vi "Get Tests for Key.vi"(8 "error in (no error)":errorcluster, 10 "Key":string, 11 "Test Event Storage in":refnum<class "Test Event Storage.lvclass">) -> (0 "error out":errorcluster, 2 "Test Events":T1[](array[typedef]), 3 "Test Event Storage out":refnum<class "Test Event Storage.lvclass">)   [LabVIEW 2009, in "Caraya.lvlib" / "Test Event Storage.lvclass"]
uses:
  Test Event Storage.lvclass
  Basic Test Manager/Assert Event Data.ctl
  Test Event Storage.lvclass/Test Event Storage.ctl
  Basic Test Manager/Basic Test Manager.lvclass
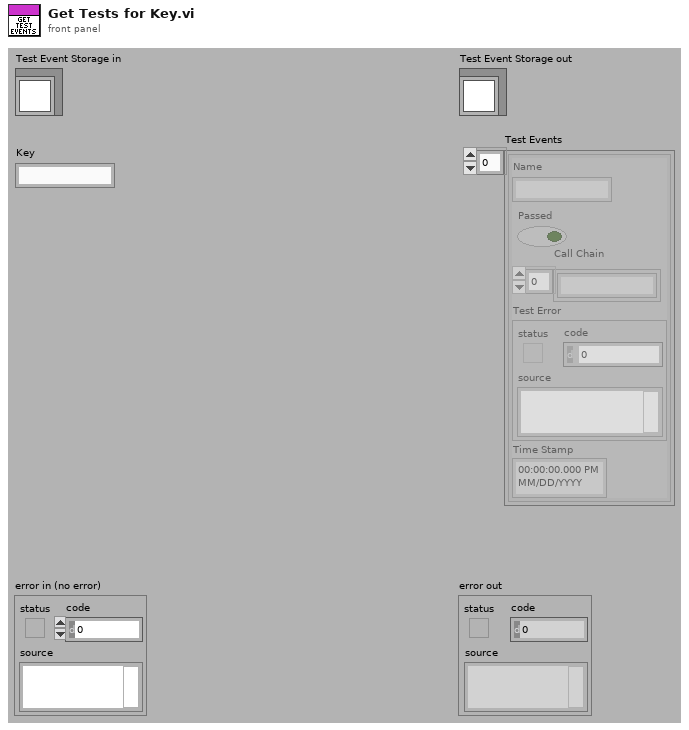
[diagram p1: front panel]
types:
  T1 = typedef "Caraya.lvlib/Basic Test Manager.lvclass/Assert Event Data.ctl" = cluster{"Name":string, "Passed":bool, "Call Chain":string[], "Test Error":errorcluster, "Time Stamp":timestamp}
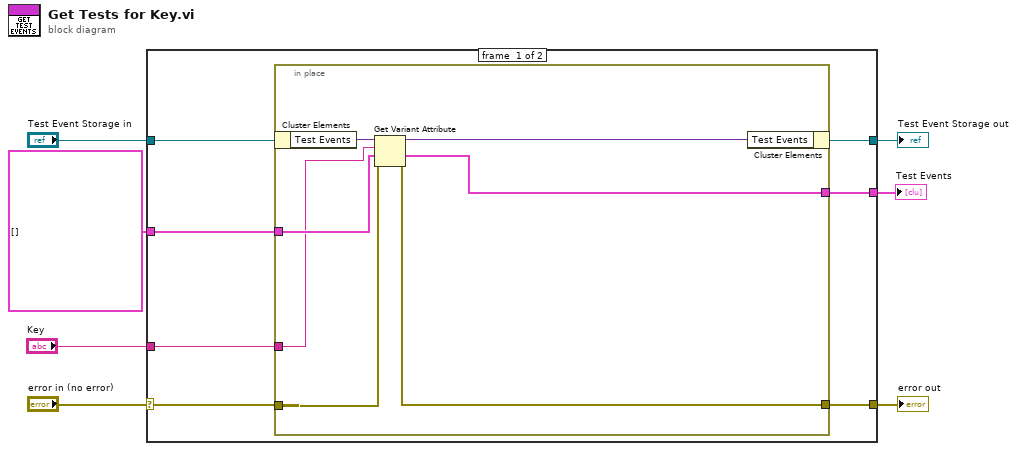
[diagram p0: block diagram]
diagram:
  n1 = case shown="No Error" "error in (no error)" {
    selector: "error in (no error)" -> [w8 w23]
    tunnel: [w14 w23] -> w6
    tunnel: [w13 w22] -> w4
    tunnel: "Test Event Storage in" -> [w10 w22]
    tunnel: T1[] [] -> [w12 _]
    tunnel: [w11 _] -> w2
    tunnel: "Key" -> [w9 _]
    frame #0 {
      n2 = in-place {
        in-place-border: w8 -> [w20]
        in-place-border: [w16] -> w14
        in-place-border: w12 -> [w18]
        in-place-border: [w17] -> w11
        in-place-border: w9 -> [w15]
        n3 = in-place-cluster #1(w10) -> ("Test Events"=w21:variant)
        n4 = Get Variant Attribute(Variant=w21, name=w15, default value (empty Variant)=w18, error in=w20) -> (duplicate Variant=w19:variant, value=w17:T1[], error out=w16:errorcluster)  [unwired: 1 out]
        n5 = in-place-cluster #1("Test Events"=w19) -> (w13:refnum<class "Test Event Storage.lvclass">)
      }
    }
    frame #1 {
    }
  }
  "error out" <- w6
  "Test Event Storage out" <- w4
  "Test Events" <- w2
